vi "Trigger State Callbacks.vi"(8 "error in (no error)":errorcluster, 10 "State":T1, 11 "Connection in":refnum<class "Connection.lvclass">) -> (0 "error out":errorcluster, 3 "Connection out":refnum<class "Connection.lvclass">)   [LabVIEW 2020, in "Stream.lvlib" / "Connection.lvclass"]
uses:
  Connection.lvclass
  C:/dev/illuminated-g/lv-stream/stream/Endpoint/Endpoint.lvclass
  Connection State.ctl
  Endpoint/Endpoint.lvclass
  Stream.lvlib
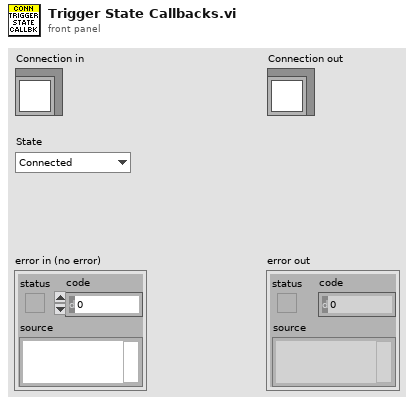
[diagram p1: front panel]
types:
  T1 = typedef "Stream.lvlib/Connection State.ctl" = enum16{"Connected", "Disconnected"}
  T2 = typedef "Stream.lvlib/Endpoint.lvclass/State Callback.ctl" = cluster{"Owner":refnum<class>, "VI":refnum<vi>, "Context":variant}
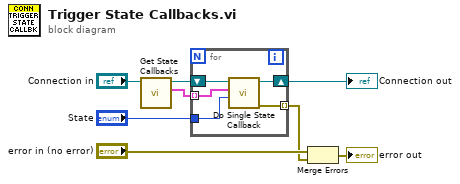
[diagram p0: block diagram]
diagram:
  n1 = call "Get State Callbacks.vi"("Endpoint in"="Connection in") -> ("State Callbacks"=w5:T2[], "Endpoint out"=w6:refnum<class "Connection.lvclass">)  [unwired: 8 in, 1 out]
  n2 = for {
    shift-right: [w9] -> w1
    shift-left: w6 -> [w13]
    tunnel: w5 -> [w12] mode=indexing
    tunnel: "State" -> [w11]
    tunnel: [w10] -> w2 mode=indexing
    n3 = call "Do Single State Callback.vi"("State"=w11, "State Callback"=w12, "Connection in"=w13) -> ("error out"=w10:errorcluster, "Connection out"=w9:refnum<class "Connection.lvclass">)  [unwired: 7 in]
  }
  "Connection out" <- w1
  n4 = Merge Errors("error in (no error)", w2) -> (→"error out":errorcluster)
